vi "Util Generate Random Value in Range.vi"(8 "error in (no error)":errorcluster, 10 "Max":dbl=1.0, 11 "Min":dbl) -> (0 "error out":errorcluster, 2 "Random Value":dbl)   [LabVIEW 2017, in "xHelper.lvlib"]
uses:
  xHelper.lvlib
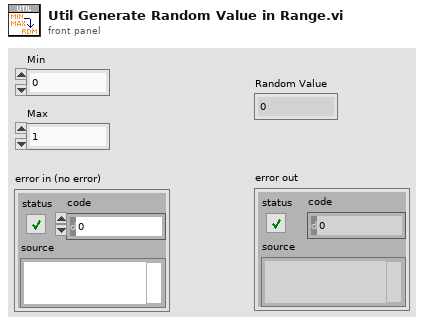
[diagram p1: front panel]
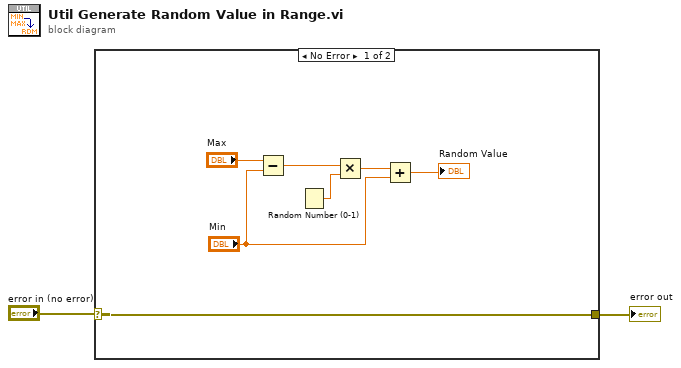
[diagram p0: block diagram]
diagram:
  n1 = case shown="No Error" "error in (no error)" {
    selector: "error in (no error)" -> [w9 w10]
    tunnel: [w9 w10] -> w1
    frame No Error {
      n2 = Subtract(x="Max", y="Min") -> (x-y=w6:dbl)
      n3 = Random Number (0-1)() -> (number: 0 to 1=w7:dbl)
      n4 = Multiply(x=w6, y=w7) -> (x*y=w5:dbl)
      n5 = Add(x=w5, y="Min") -> (x+y=→"Random Value":dbl)
    }
    frame Error {
    }
  }
  "error out" <- w1
